vi "DynamicCallVI-Not Open Frant Panel.vi"(8 "error in (no error)":errorcluster, 10 "name or relative path":string, 11 "base path":path) -> (0 "error out":errorcluster)   [LabVIEW 2021]
doc: "dynamic call a vi, is used in the launcher, usually.\nNot open frant panel.\n2015-03-03 16:23:16\n蒋松\njiangsong@outlook.com"
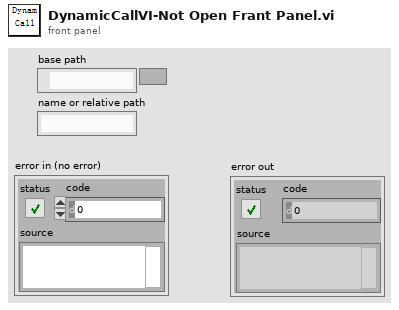
[diagram p1: front panel]
types:
  T1 = enum32{"Invalid", "Standard", "Closed", "Hidden", "Minimized", "Maximized"}
  T2 = enum32{"Bad", "Idle", "Run top level", "Running"}
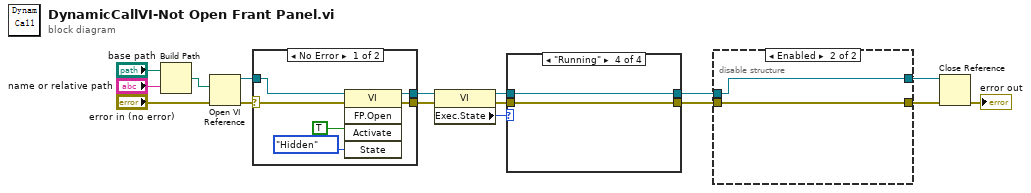
[diagram p0: block diagram]
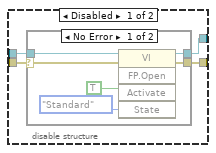
[diagram p2: hidden frame]
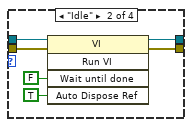
[diagram p5: hidden frame]
diagram:
  n1 = Build Path(base path="base path", name or relative path="name or relative path") -> (appended path=w16:path)
  n2 = Open VI Reference(vi path=w16, error in (no error)="error in (no error)") -> (vi reference=w14:refnum<vi>, error out=w15:errorcluster)  [unwired: 4 in]
  n3 = case shown="No Error" w15 {
    selector: w15 -> [w17 w23]
    tunnel: [w20 w23] -> w13
    tunnel: w14 -> [w19 w24]
    tunnel: [w18 w24] -> w9
    frame No Error {
      n4 = invoke class="VI" method="FP.Open"(reference=w19, error in=w17, "Activate"=TRUE, "State"=T1."Hidden") -> (reference out=w18:refnum<vi>, error out=w20:errorcluster)  [unwired: 1 in, 3 out]
    }
    frame Error {
    }
  }
  n5 = property class="VI"(reference=w9, error in=w13) -> (reference out=w11:refnum<vi>, error out=w10:errorcluster, "Exec.State"=w12:T2)
  n6 = case shown="\"Running\"" w12 {
    tunnel: w11 -> [w26 w30 w34 w36]
    tunnel: w10 -> [w25 w29 w33 w35]
    tunnel: [w26 w28 w34 w36] -> w8
    tunnel: [w25 w27 w33 w35] -> w6
    frame "Bad", Default {
    }
    frame "Idle" {
      n7 = invoke class="VI" method="Run VI"(reference=w30, error in=w29, "Wait until done"=FALSE ("Wait Until Done"), "Auto Dispose Ref"=TRUE ("Auto Dispose Reference")) -> (reference out=w28:refnum<vi>, error out=w27:errorcluster)  [unwired: 1 in, 3 out]
    }
    frame "Run top level" {
    }
    frame "Running" {
    }
  }
  n8 = disable-structure shown="Enabled" {
    disable-tunnel: w8 -> [w40 w50]
    disable-tunnel: [w39 w50] -> w7
    disable-tunnel: w6 -> [w38 w49]
    disable-tunnel: [w37 w49] -> w5
    frame Disabled {
      n9 = case shown="No Error" w38 {
        selector: w38 -> [w41 w47]
        tunnel: [w44 w47] -> w37
        tunnel: w40 -> [w43 w48]
        tunnel: [w42 w48] -> w39
        frame No Error {
          n10 = invoke class="VI" method="FP.Open"(reference=w43, error in=w41, "Activate"=TRUE, "State"=T1."Standard") -> (reference out=w42:refnum<vi>, error out=w44:errorcluster)  [unwired: 1 in, 3 out]
        }
        frame Error {
        }
      }
    }
    frame Enabled {
    }
  }
  n11 = Close Reference(reference=w7, error in (no error)=w5) -> (error out=→"error out":errorcluster)
